vi "SecondaryData_Position.vi"(9 "Variant":variant, 10 "Input":dbl[](array[numeric]), 11 "Option":i32) -> (2 "SecondaryData":dbl[](array[numeric]))   [LabVIEW 2013]
uses:
  <instrlib>/ESP300/Public/Position_ESP300.vi
  <instrlib>/Micos_uic/Public/Position_Micos.vi
  <instrlib>/ESP300/ESP300.lvlib
  <instrlib>/Micos_uic/Micos_uic.lvlib
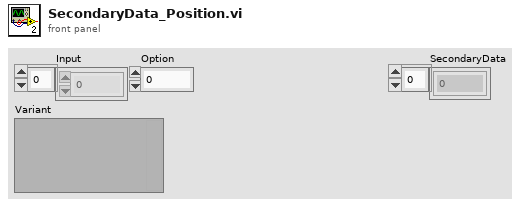
[diagram p1: front panel]
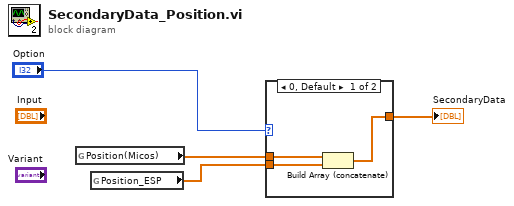
[diagram p0: block diagram]
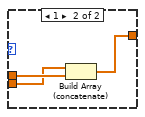
[diagram p2: hidden frame]
diagram:
  n1 = global read "Position_Micos.vi" "Position(Micos)"() -> (w4:dbl[])
  n2 = global read "Position_ESP300.vi" "Position_ESP"() -> (w3:dbl[])
  n3 = case shown="0, Default" "Option" {
    tunnel: w4 -> [w7 w10]
    tunnel: w3 -> [w6 w9]
    tunnel: [w5 w8] -> w2
    frame 0, Default {
      n4 = Build Array (concatenate)(w7, w6) -> (w5:dbl[])
    }
    frame 1 {
      n5 = Build Array (concatenate)(w9, w10) -> (w8:dbl[])
    }
  }
  "SecondaryData" <- w2
